vi "ErrorReport.vi"(8 "error in (no error)":errorcluster, 11 "Source":string) -> ()   [LabVIEW 2013]
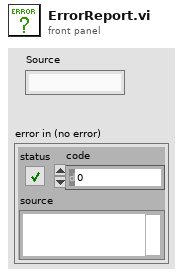
[diagram p1: front panel]
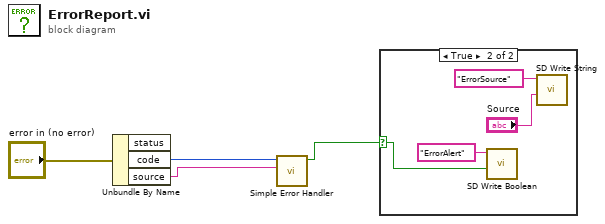
[diagram p0: block diagram]
diagram:
  n1 = Unbundle By Name("error in (no error)") -> ("code"=w2:i32, "source"=w3:string)  [unwired: 1 out]
  n2 = call <vilib>:"Simple Error Handler.vi"("error code (no error:0)"=w2, "error source (\" \")"=w3) -> ("error?"=w1:bool)  [unwired: 3 in, 4 out]
  n3 = case shown="True" w1 {
    selector: w1 -> [_ w5]
    frame False {
    }
    frame True {
      n4 = call <vilib>:"SD Write Boolean.vi"("Boolean"=w5, "Name"="ErrorAlert") -> ()  [unwired: 8 in, 2 out]
      n5 = call <vilib>:"SD Write String.vi"("String"="Source", "Name"="ErrorSource") -> ()  [unwired: 8 in, 2 out]
    }
  }
